vi "main.vi"() -> ()   [LabVIEW 2021]
uses:
  <vilib>/Platform/TimedLoop/XDataNode/timing_clust.ctl
  <vilib>/Platform/TimedLoop/XDataNode/nitl_modes.ctl
  <vilib>/Platform/TimedLoop/XDataNode/wakeup.ctl
  <vilib>/platform/TimedLoop/XDataNode/XDataNode.xnode
  <vilib>/Platform/TimedLoop/XDataNode/XDNodeRunTimeDep.lvlib
panel:
  out "pictureOut":picture
  out "ArrayOut":bool[][](array[boolean])
  out "error out":errorcluster
  in  "stop":bool
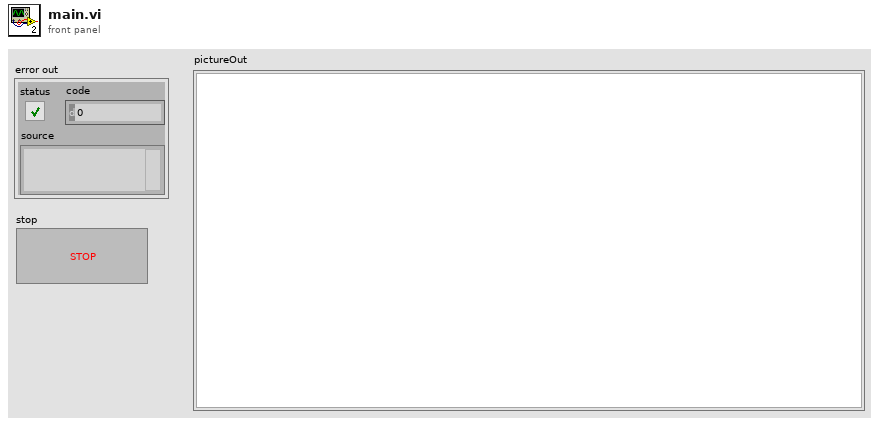
[diagram p1: front panel]
types:
  T1 = typedef "XDNodeRunTimeDep.lvlib/timing_clust.ctl" = cluster{"Expected End [f-1]":u64, "Actual End [f-1]":u64, "Finished Late? [f-1]":bool, "Expected End [i-1]":u64, "Actual End [i-1]":u64, "Finished Late? [i-1]":bool, "Expected Start [i]":u64, "Actual Start [i]":u64, "Expected Start [f]":u64, "Actual Start [f]":u64, "Source Name":string, "Structure Name":string, "Period":i64, "Deadline":i64, "Offset":i64, "Start":i64, "Priority":i32, "Timeout":i32, "Mode":T2, "Wakeup Reason":T3, "Error":errorcluster, "Source Type":string, "Secondary Source Type":string, "Global End Time":u64, "Global Start Time":u64, "Frame Duration":u64, "Iteration Duration":u64, "Assigned CPU":i32, "I/O Scan Engine Mode":u32}
  T2 = typedef "XDNodeRunTimeDep.lvlib/nitl_modes.ctl" = enum32{"No Change", "Process missed periods, maintain original phase", "Discard missed periods, maintain original phase", "Process missed periods, ignore original phase", "Discard missed periods, ignore original phase"}
  T3 = typedef "XDNodeRunTimeDep.lvlib/wakeup.ctl" = enum32{"Normal", "Aborted", "Asynchronous wakeup", "Timing source error", "Timed loop error", "Timeout"}
  T4 = enum16{"Standard", "Buffered", "CRLF", "Immediate"}
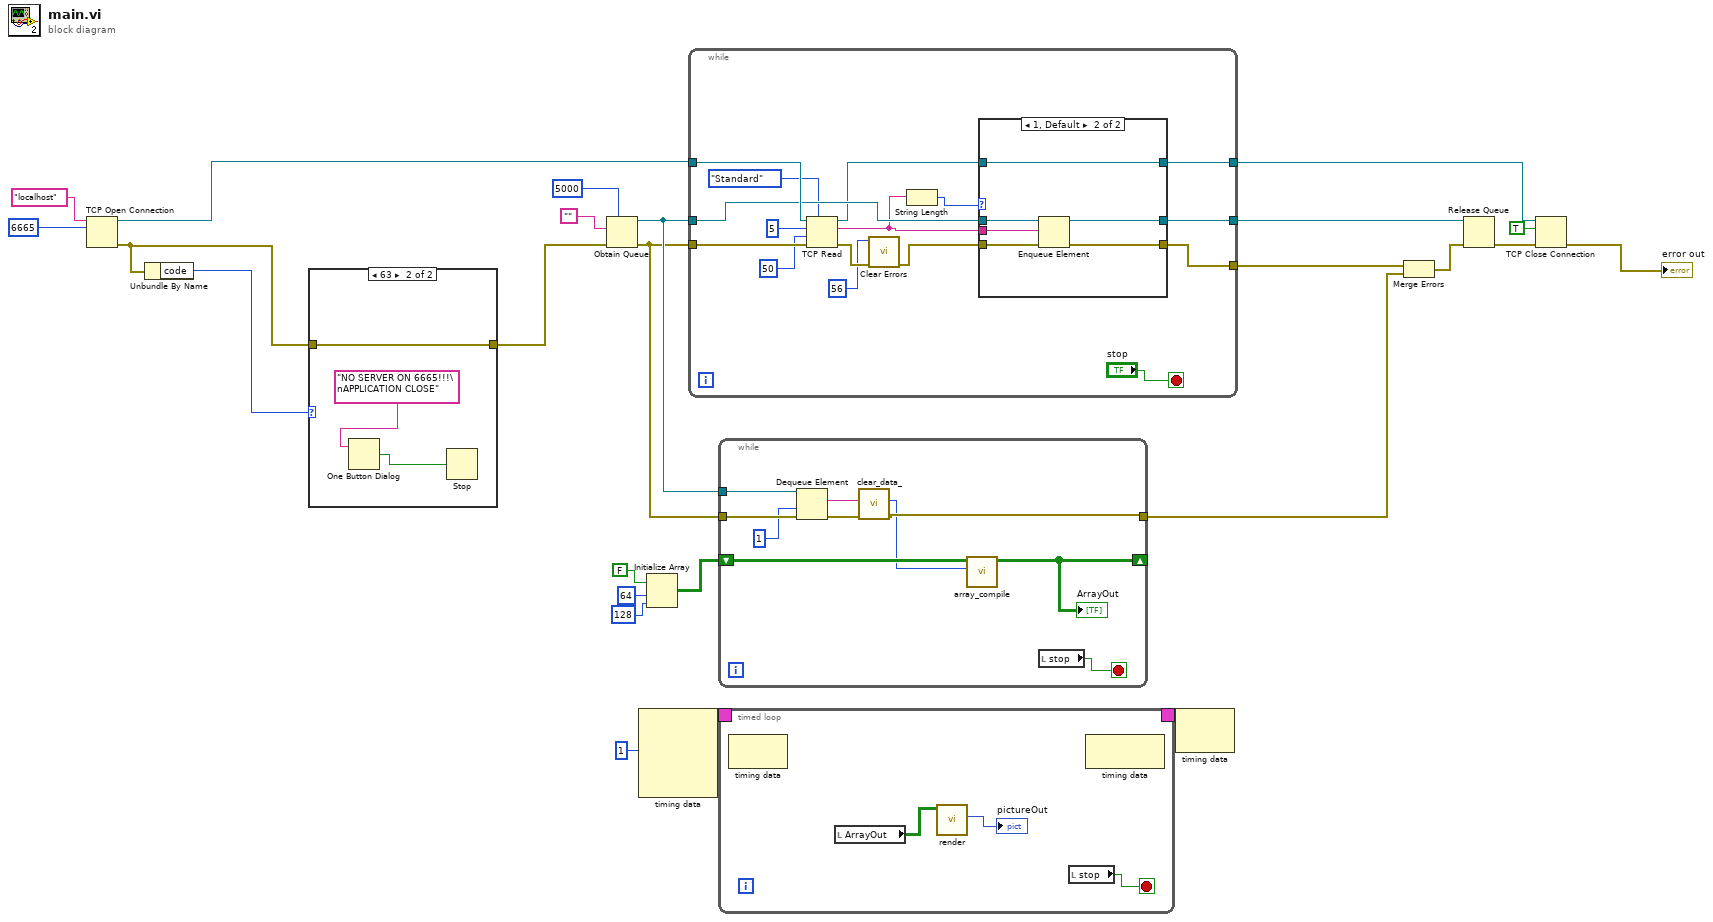
[diagram p0: block diagram]
diagram:
  n1 = TCP Open Connection(address="localhost", remote port or service name=u16 6665 ("local port (0)")) -> (connection ID=w25:refnum<k5>, error out=w3:errorcluster)  [unwired: 3 in]
  n2 = Unbundle By Name(w3) -> ("code"=w2:i32)
  n3 = case shown="63" w2 {
    tunnel: w3 -> [w26 w27]
    tunnel: [w26 w27] -> w1
    frame 0, Default {
    }
    frame 63 {
      n4 = One Button Dialog(message="NO SERVER ON 6665!!!\nAPPLICATION CLOSE") -> (true=w28:bool)  [unwired: 1 in]
      n5 = Stop(stop? (T)=w28) -> ()
    }
  }
  n6 = Obtain Queue(max queue size (-1, unlimited)=5000, element data type="", error in (no error)=w1) -> (queue out=w19:refnum<queue>, error out=w18:errorcluster)  [unwired: 2 in, 1 out]
  n7 = node-c288(i64 1 ("Period")) -> (w8:T1)  [unwired: 3 in]
  n8 = Initialize Array(FALSE, 64 ("dimension size"), 128 ("dimension size")) -> (w9:bool[][])
  n9 = while {
    tunnel: w25 -> [w43]
    tunnel: [w31] -> w24
    tunnel: w18 -> [w45]
    tunnel: w19 -> [w42]
    tunnel: [w37] -> w16
    tunnel: [w41] -> w23
    stop <- "stop" stop-if-true
    n10 = TCP Read(connection ID=w43, bytes to read=5, error in (no error)=w45, 7:T4."Standard" ("mode (standard)"), 9:50 ("timeout ms (25000)")) -> (connection ID out=w32:refnum<k5>, data out=w34:string, error out=w40:errorcluster)
    n11 = call <vilib>:"Clear Errors.vi"("error in (no error)"=w40, "specific error code to clear (0: all)"=56) -> ("error out"=w38:errorcluster)  [unwired: 4 in, 1 out]
    n12 = String Length(string=w34) -> (length=w33:i32)
    n13 = case shown="1, Default" w33 {
      tunnel: w42 -> [w48 w54]
      tunnel: [w48 w53] -> w41
      tunnel: w38 -> [w47 w52]
      tunnel: [w47 w50] -> w37
      tunnel: w34 -> [_ w51]
      tunnel: w32 -> [w46 w49]
      tunnel: [w46 w49] -> w31
      frame 0 {
      }
      frame 1, Default {
        n14 = Enqueue Element(queue=w54, element=w51, error in (no error)=w52) -> (queue out=w53:refnum<queue>, error out=w50:errorcluster)  [unwired: 1 in, 1 out]
      }
    }
  }
  n15 = while {
    tunnel: w19 -> [w64]
    tunnel: w18 -> [w63]
    tunnel: [w56] -> w15
    shift-right: [w61] -> _
    shift-left: w9 -> [w62]
    stop <- w59 stop-if-true
    n16 = Dequeue Element(queue=w64, timeout in ms (-1)=1, error in (no error)=w63) -> (element=w58:string, error out=w57:errorcluster)  [unwired: 2 out]
    n17 = call "clear_data_.vi"("error in (no error)"=w57, "dataIn"=w58) -> ("error out"=w56:errorcluster, "dataOut"=w55:u32)  [unwired: 6 in]
    n18 = call "array_compile.vi"("dataIn"=w55, "ArrayIn"=w62) -> ("ArrayOut"=w61:bool[][])  [unwired: 9 in]
    "ArrayOut" <- w61
    n19 = local read "stop"() -> (w59:bool)
  }
  n20 = timed-loop {
    timing: w8 -> [_]
    timing-out: [_] -> w7
    stop <- w67 stop-if-true
    n21 = node-c288() -> ()  [unwired: 1 in, 1 out]
    n22 = local read "ArrayOut"() -> (w66:bool[][])
    n23 = call "render.vi"("ArrayIn"=w66) -> ("pictureOut"=→"pictureOut":picture)  [unwired: 10 in]
    n24 = local read "stop"() -> (w67:bool)
    n25 = node-c288() -> ()  [unwired: 1 in, 1 out]
  }
  n26 = node-c288(w7) -> ()  [unwired: 1 out]
  n27 = Merge Errors(w16, w15) -> (w14:errorcluster)
  n28 = Release Queue(queue=w23, error in (no error)=w14) -> (error out=w22:errorcluster)  [unwired: 1 in, 2 out]
  n29 = TCP Close Connection(connection ID=w24, abort (F)=TRUE, error in (no error)=w22) -> (error out=→"error out":errorcluster)  [unwired: 1 out]
